vi "Initialize.vi"(2 "IP address":string="192.168.4.129", 5 "error in":errorcluster) -> (14 "RedPitaya connection out":refnum<k5>, 19 "error out":errorcluster)   [LabVIEW 2021, in "RedPitaya.lvlib"]
doc: "Establishes communication with Red Pitaya. Generally, you need to call the Initialize VI only once at the beginning of an application."
uses:
  RedPitaya.lvlib
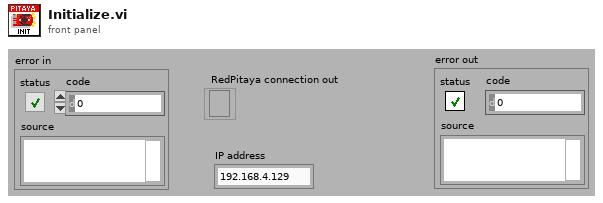
[diagram p1: front panel]
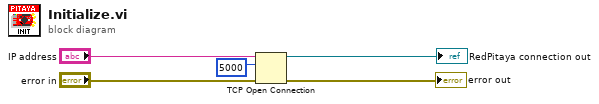
[diagram p0: block diagram]
diagram:
  n1 = TCP Open Connection(address="IP address", remote port or service name=u16 5000, error in (no error)="error in") -> (connection ID=→"RedPitaya connection out":refnum<k5>, error out=→"error out":errorcluster)  [unwired: 2 in]
